vi "unload.vi"(8 "error in (no error)":errorcluster, 10 "pdbm_taskroute_reg_event":T2, 11 "pdbm_taskroute_event":T1) -> (0 "error out":errorcluster, 3 "pdbm_testsys_fd_event":refnum<user-event>)   [LabVIEW 2015, in "pdbm_task_route.lvlib"]
uses:
  pdbm_task_route.lvlib
  test_system/UsrDefine/pdbm_testsystem_feedback_data.ctl
  pdbm_testsys_taskroute_inter/UsrDefine/pdbm_testsys_reqst_data.ctl
  UsrDefine/TaskFeedbackCmd.ctl
  pdbm_testsys_taskroute_inter/pdbm_testsys_taskroute_inter.lvlib
  test_system/pdbm_test_system.lvlib
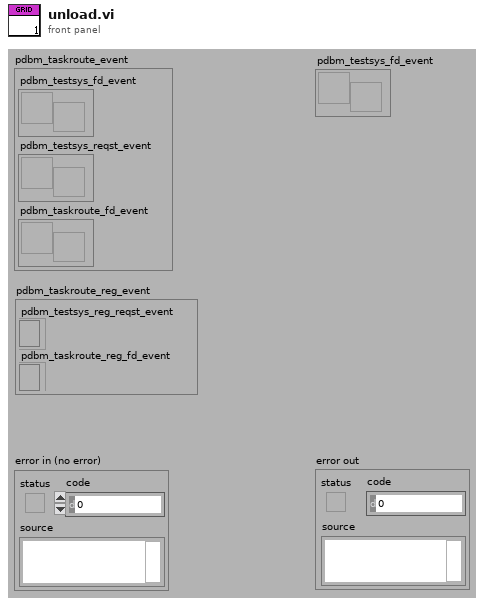
[diagram p1: front panel]
types:
  T1 = cluster{"pdbm_testsys_fd_event":refnum<user-event>, "pdbm_testsys_reqst_event":refnum<user-event>, "pdbm_taskroute_fd_event":refnum<user-event>}
  T2 = cluster{"pdbm_testsys_reg_reqst_event":refnum<event-registration>, "pdbm_taskroute_reg_fd_event":refnum<event-registration>}
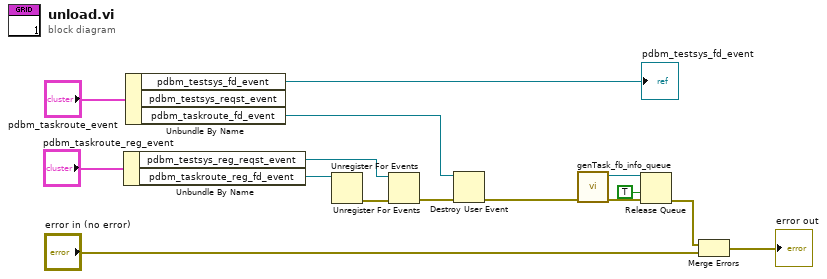
[diagram p0: block diagram]
diagram:
  n1 = Unbundle By Name("pdbm_taskroute_reg_event") -> ("pdbm_testsys_reg_reqst_event"=w12:refnum<event-registration>, "pdbm_taskroute_reg_fd_event"=w14:refnum<event-registration>)
  n2 = Unbundle By Name("pdbm_taskroute_event") -> ("pdbm_testsys_fd_event"=→"pdbm_testsys_fd_event":refnum<user-event>, "pdbm_taskroute_fd_event"=w2:refnum<user-event>)  [unwired: 1 out]
  n3 = Unregister For Events(event registration refnum=w14) -> (error out=w13:errorcluster)  [unwired: 1 in]
  n4 = Unregister For Events(event registration refnum=w12, error in=w13) -> (error out=w3:errorcluster)
  n5 = Destroy User Event(user event=w2, error in=w3) -> (error out=w1:errorcluster)
  n6 = call "genTask_fb_info_queue.vi"("error in (no error)"=w1) -> ("error IO"=w10:errorcluster, "pdbm_task_fb_info_queue"=w9:refnum<queue>)  [unwired: 9 in]
  n7 = Release Queue(queue=w9, force destroy? (F)=TRUE, error in (no error)=w10) -> (error out=w7:errorcluster)  [unwired: 2 out]
  n8 = Merge Errors(w7, "error in (no error)") -> (→"error out":errorcluster)
